vi "Double 1D to Data Type.vi"(8 "error in (no error)":errorcluster, 11 "Boolean 1D":dbl[](array[numeric])) -> (0 "error out":errorcluster, 3 "Boolean out":refnum<class "Double 1D.lvclass">)   [LabVIEW 2020, in "Double 1D.lvclass"]
uses:
  <vilib>/gpm_packages/@cs/data-type-serializer/source/Double 1D/Double 1D.lvclass
  <vilib>/gpm_packages/@cs/data-type-serializer/source/Double 1D/Double 1D.lvclass/Double 1D.ctl
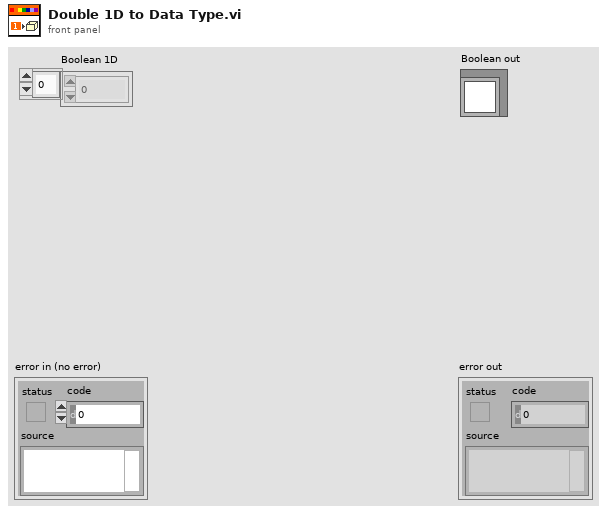
[diagram p1: front panel]
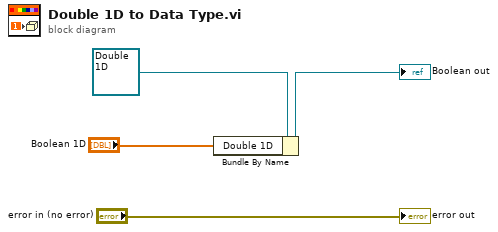
[diagram p0: block diagram]
diagram:
  n1 = Bundle By Name(cluster=refnum<class "Double 1D.lvclass"> refnum ("Boolean in"), "Double 1D"="Boolean 1D") -> (→"Boolean out":refnum<class "Double 1D.lvclass">)
  "error out" <- "error in (no error)"
